vi "ex4.vi"() -> ()   [LabVIEW 2022 SP3]
panel:
  in  "Stop Button":bool
  out "Seconds":i32
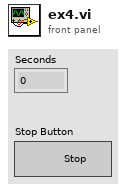
[diagram p1: front panel]
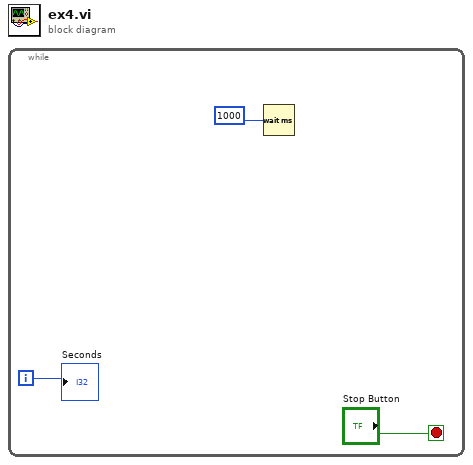
[diagram p0: block diagram]
diagram:
  n1 = while {
    i -> [w2]
    stop <- "Stop Button" stop-if-true
    n2 = Wait (ms)(milliseconds to wait=1000) -> ()  [unwired: 1 out]
    "Seconds" <- w2
  }
